vi "ILC J1-19.vi"(8 "error":errorcluster, 11 "VISA":refnum<visa-resource-name>) -> (0 "error out":errorcluster, 3 "VISA out":refnum<visa-resource-name>)   [LabVIEW 2023, in "TDK20-38 API.lvlib"]
uses:
  TDK20-38 API.lvlib
  <userlib>/TDK-Lambda GEN LAN Series/TDK-Lambda GEN LAN Series.lvlib
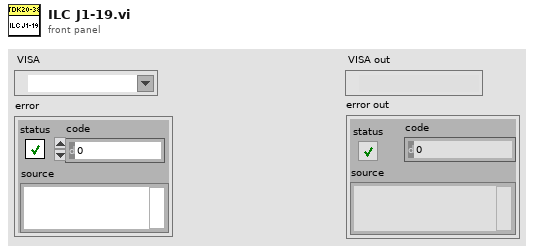
[diagram p1: front panel]
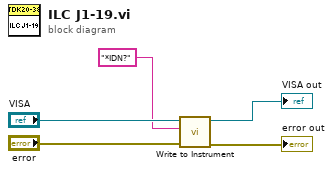
[diagram p0: block diagram]
diagram:
  n1 = call <userlib>:"Write to Instrument.vi"("error"="error", "Command"="*IDN?" ("format string"), "VISA"="VISA") -> ("error out"=→"error out":errorcluster, "VISA out"=→"VISA out":refnum<visa-resource-name>)  [unwired: 7 in]
